vi "Polling Verse Event Driven Code.vi"() -> ()   [LabVIEW 2020]
panel:
  out "x+y":dbl
  in  "y":dbl
  in  "x":dbl
  out "a+b":dbl
  in  "a":dbl
  in  "b":dbl
  out "Iteration Count - Event":i32
  out "Iteration Count - Polling":i32
  in  "stop":bool
  # "Polling"
  # "Event"
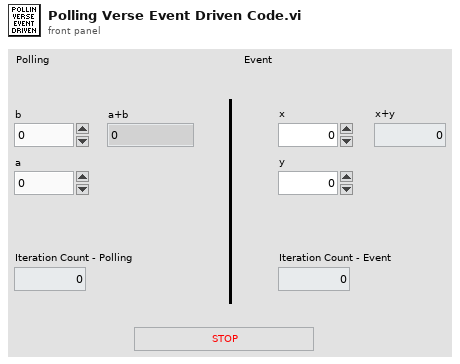
[diagram p1: front panel]
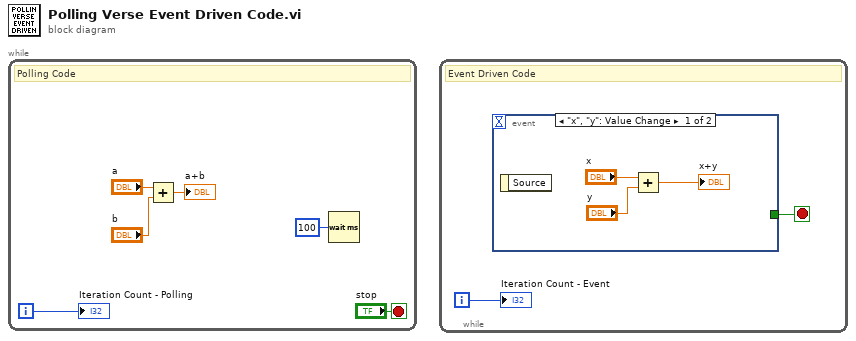
[diagram p0: block diagram]
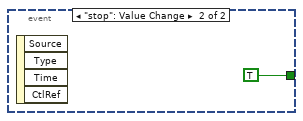
[diagram p2: hidden frame]
diagram:
  n1 = while {
    i -> [w5]
    stop <- "stop" stop-if-true
    # "Polling Code"
    n2 = Add(x="a", y="b") -> (x+y=→"a+b":dbl)
    n3 = Wait (ms)(milliseconds to wait=u32 100) -> ()  [unwired: 1 out]
    "Iteration Count - Polling" <- w5
  }
  n4 = while {
    i -> [w8]
    stop <- w7 stop-if-true
    # "Event Driven Code"
    n5 = event shown="[0] \"x\", \"y\": Value Change" {
      selector: _ -> [_ _]
      dyn-events: _ -> [_ _]
      timeout: _ -> [_ _]
      tunnel: [_ TRUE] -> w7
      event "x", "y": Value Change {
        n6 = event-data() -> ()  [unwired: 1 in, 1 out]
        n7 = Add(x="x", y="y") -> (x+y=→"x+y":dbl)
      }
      event "stop": Value Change {
        n8 = event-data() -> ()  [unwired: 1 in, 4 out]
      }
    }
    "Iteration Count - Event" <- w8
  }
